vi "parse_GPGGA.vi"(0 "NMEA GPGGA String":string) -> (2 "Valid GPS Fix?":bool, 3 "Time":string, 4 "GPS Coordinate":T1 {"Elev. (m)" format="%_12g"; "Lon (deg)" format="%_12g"; "Lat (deg)" format="%_12g"}, 5 "nSatellites":i32, 6 "HDOP":dbl)   [LabVIEW 2010]
doc: "Pass this VI an NMEA sentence and it will parse it as if it's a GPGGA sentence.\nThe Valid GPS output will be false if there's no fix or if it's not a GPGGA sentence."
uses:
  _typedefs/GPS Coordinate.ctl
panel:
  out "$GPGGA Code":string
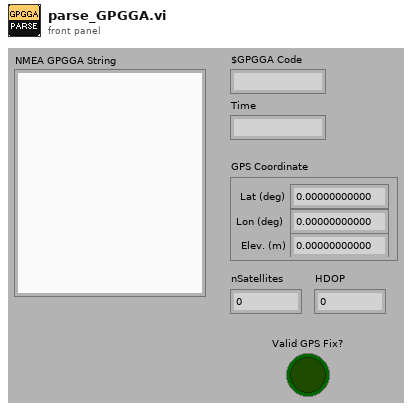
[diagram p1: front panel]
types:
  T1 = typedef "GPS Coordinate.ctl" = cluster{"Lat (deg)":dbl, "Lon (deg)":dbl, "Elev. (m)":dbl}
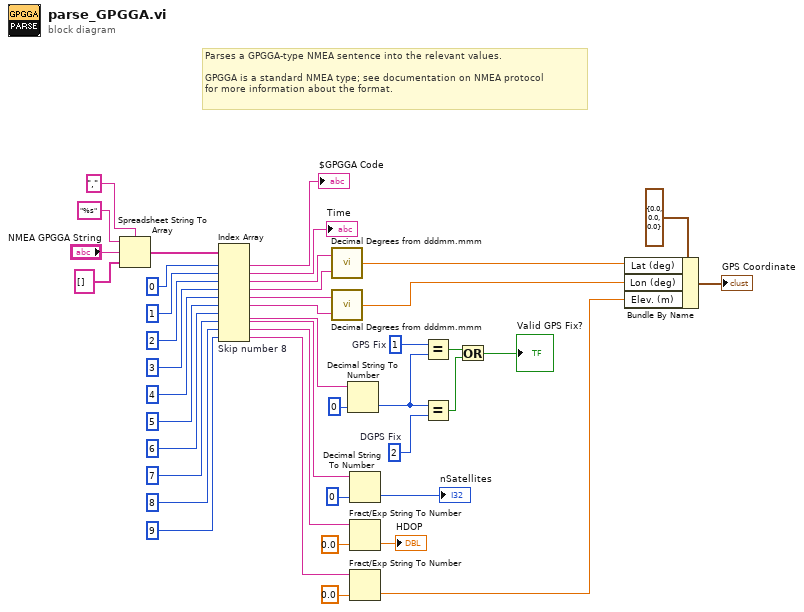
[diagram p0: block diagram]
diagram:
  w40 = 2  # DGPS Fix
  w3 = 1  # GPS Fix
  # "Parses a GPGGA-type NMEA sentence into the relevant values.\n\nGPGGA is a standard NMEA type; see documentation on NMEA protocol\nfor more information about the format."
  n1 = Spreadsheet String To Array(delimiter (Tab)=",", format string="%s", spreadsheet string="NMEA GPGGA String", array type (2D Dbl)=string[] []) -> (array=w35:string[])
  n2 = Index Array "Skip number 8"(array=w35, index #1=0 ("index"), index #2=1 ("index"), index #3=2 ("index"), index #4=3 ("index"), index #5=4 ("index"), index #6=5 ("index"), index #7=6 ("index"), index #8=7 ("index"), index #9=8 ("index"), index #10=9 ("index")) -> (element #1=→"$GPGGA Code":string, element #2=→"Time":string, element #3=w31:string, element #4=w30:string, element #5=w29:string, element #6=w28:string, element #7=w27:string, element #8=w26:string, element #9=w25:string, element #10=w9:string)
  n3 = call "Decimal Degrees from dddmm.mmm.vi"("Hemisphere Letter"=w30, "Degrees String"=w31) -> ("Decimal Degrees"=w8:dbl)
  n4 = call "Decimal Degrees from dddmm.mmm.vi"("Hemisphere Letter"=w28, "Degrees String"=w29) -> ("Decimal Degrees"=w7:dbl)
  n5 = Decimal String To Number(string=w27, default (0L)=0) -> (number=w4:i32)  [unwired: 2 out]
  n6 = Decimal String To Number(string=w26, default (0L)=0) -> (number=→"nSatellites":i32)  [unwired: 2 out]
  n7 = Fract/Exp String To Number(string=w25, default (0 dbl)=0.0) -> (number=→"HDOP":dbl)  [unwired: 2 in, 1 out]
  n8 = Fract/Exp String To Number(string=w9, default (0 dbl)=0.0) -> (number=w6:dbl)  [unwired: 2 in, 1 out]
  n9 = Equal?(x=w3, y=w4) -> (x = y?=w16:bool)
  n10 = Equal?(x=w4, y=w40) -> (x = y?=w17:bool)
  n11 = Or(x=w16, y=w17) -> (x .or. y?=→"Valid GPS Fix?":bool)
  n12 = Bundle By Name(cluster=T1 {"Lat (deg)"=0.0, "Lon (deg)"=0.0, "Elev. (m)"=0.0} ("GPS Coordinate"), "Lat (deg)"=w8, "Lon (deg)"=w7, "Elev. (m)"=w6) -> (→"GPS Coordinate":T1)
